vi "Close Note File.vi"(8 "Error In":errorcluster, 10 "Notes":string, 11 "file path":path) -> (0 "Error Out":errorcluster)   [LabVIEW 2018]
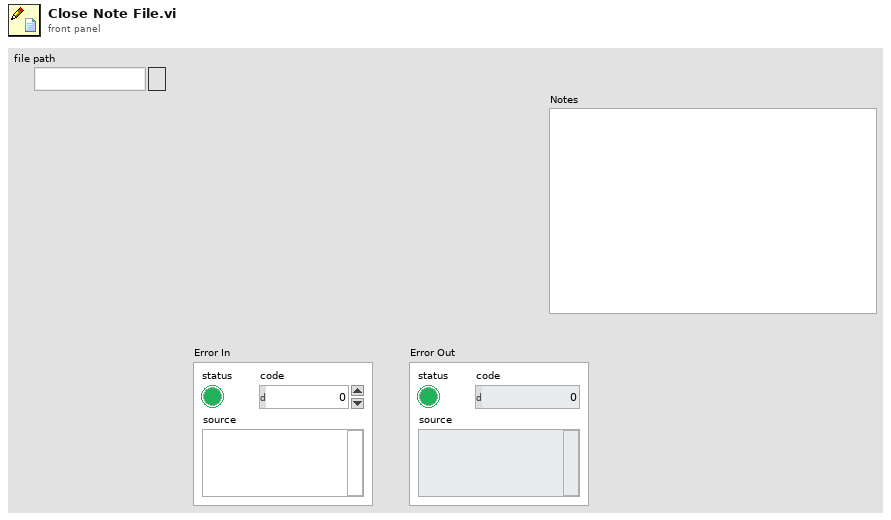
[diagram p1: front panel]
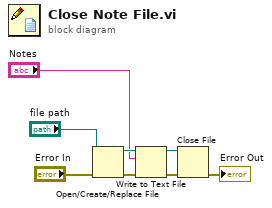
[diagram p0: block diagram]
diagram:
  n1 = Open/Create/Replace File(file path (use dialog)="file path", error in="Error In") -> (refnum out=w8:refnum<file>, error out=w7:errorcluster)  [unwired: 4 in, 1 out]
  n2 = Write to Text File(file (use dialog)=w8, text="Notes", error in=w7) -> (refnum out=w6:refnum<file>, error out=w3:errorcluster)  [unwired: 1 in, 1 out]
  n3 = Close File(refnum=w6, error in=w3) -> (error out=→"Error Out":errorcluster)  [unwired: 1 out]
